vi "Add Subscriber to List.vi"(10 "Subscription":T1, 11 "MVC Subscription in":refnum<class "MVC Subscription.lvclass">) -> (3 "MVC Subscription out":refnum<class "MVC Subscription.lvclass">)   [LabVIEW 2014, in "MVC Subscription.lvlib" / "MVC Subscription.lvclass"]
uses:
  MVC Subscription.lvclass
  Cluster - Individual Subscription.ctl
  <vilib>/ActorFramework/Message Enqueuer/Message Enqueuer.lvclass
  <vilib>/ActorFramework/Message/Message.lvclass
  MVC Subscription.lvclass/MVC Subscription.ctl
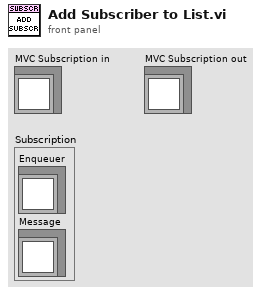
[diagram p1: front panel]
types:
  T1 = typedef "MVC Subscription.lvlib/MVC Subscription.lvclass/Cluster - Individual Subscription.ctl" = cluster{"Enqueuer":refnum<class "Message Enqueuer.lvclass">, "Message":refnum<class "Message.lvclass">}
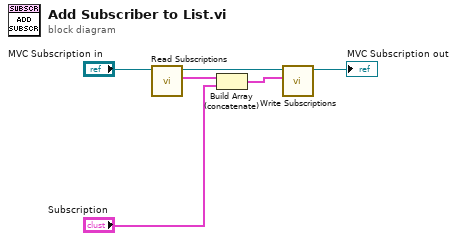
[diagram p0: block diagram]
diagram:
  n1 = call "Read Subscriptions.vi"("MVC Subscription in"="MVC Subscription in") -> ("Subscriptions"=w3:T1[], "MVC Subscription out"=w1:refnum<class "MVC Subscription.lvclass">)  [unwired: 9 in]
  n2 = Build Array (concatenate)(w3, "Subscription") -> (w5:T1[])
  n3 = call "Write Subscriptions.vi"("Subscriptions"=w5, "MVC Subscription in"=w1) -> ("MVC Subscription out"=→"MVC Subscription out":refnum<class "MVC Subscription.lvclass">)  [unwired: 9 in]
